vi "General Format query.vi"() -> ()   [LabVIEW 2009]
panel:
  in  "VISA resource name":refnum<visa-resource-name>="GPIB0::21::INSTR"
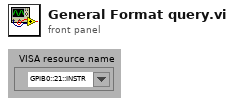
[diagram p1: front panel]
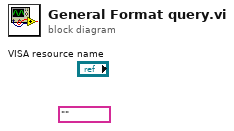
[diagram p0: block diagram]
diagram:
  (unwired) ""
